vi "1D_2D.vi"(11 "Array_IN":u32[](array[colorbox])=[15463629, 16769393, 2837841, 16753544, 10003068]) -> (3 "Array_Out":u32[][](array[numeric]))   [LabVIEW 2017]
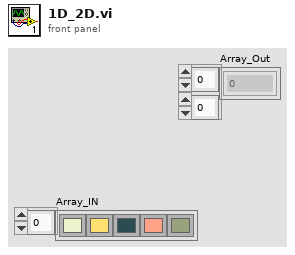
[diagram p1: front panel]
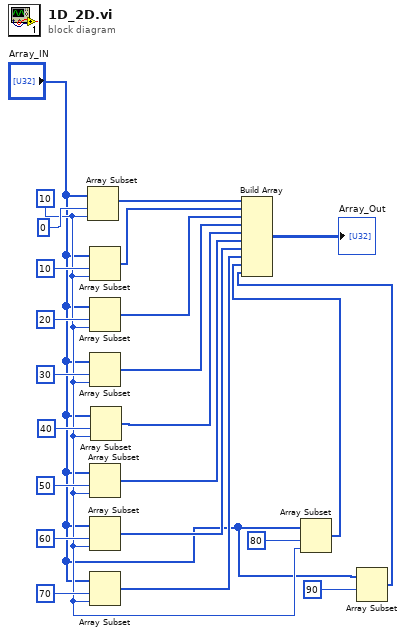
[diagram p0: block diagram]
diagram:
  w12 = 10 ("length")
  n1 = Array Subset "Array Subset"(array="Array_IN", index=0 ("length"), length=w12) -> (w23:u32[])
  n2 = Array Subset "Array Subset"(array="Array_IN", index=10, length=w12) -> (w21:u32[])
  n3 = Array Subset "Array Subset"(array="Array_IN", index=20, length=w12) -> (w11:u32[])
  n4 = Array Subset "Array Subset"(array="Array_IN", index=30, length=w12) -> (w10:u32[])
  n5 = Array Subset "Array Subset"(array="Array_IN", index=50, length=w12) -> (w8:u32[])
  n6 = Array Subset "Array Subset"(array="Array_IN", index=60, length=w12) -> (w7:u32[])
  n7 = Array Subset "Array Subset"(array="Array_IN", index=70, length=w12) -> (w6:u32[])
  n8 = Array Subset "Array Subset"(array="Array_IN", index=40, length=w12) -> (w9:u32[])
  n9 = Array Subset "Array Subset"(array="Array_IN", index=80, length=w12) -> (w5:u32[])
  n10 = Array Subset "Array Subset"(array="Array_IN", index=90) -> (w3:u32[])  [unwired: 1 in]
  n11 = Build Array(w23, w21, w11, w10, w9, w8, w7, w6, w5, w3) -> (→"Array_Out":u32[][])
